vi "Init.vi"(8 "error in (no error)":errorcluster, 9 "Clock type":enum8{"Internal", "External", "PXI"}(ring), 10 "Slot":u16) -> (0 "error out":errorcluster, 3 "MagiQmw3 out":refnum<class "MagiQmw3.lvclass">)   [LabVIEW 2010, in "MagiQmw3.lvclass"]
uses:
  MagiQmw3.lvclass
panel:
  out "path":path
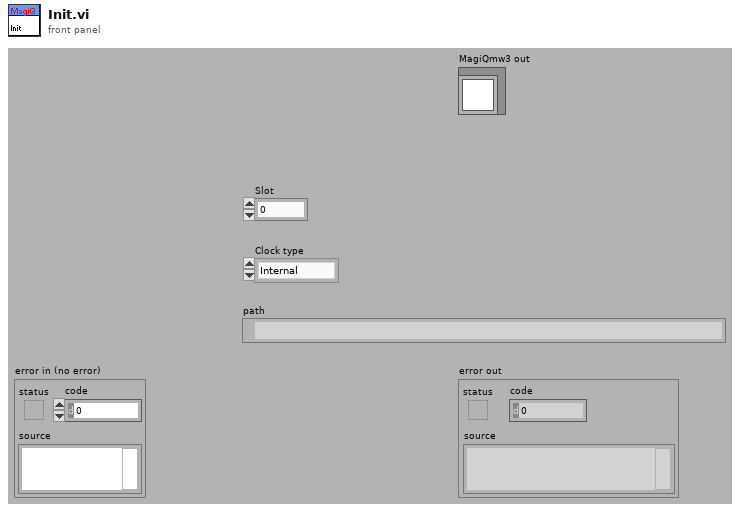
[diagram p1: front panel]
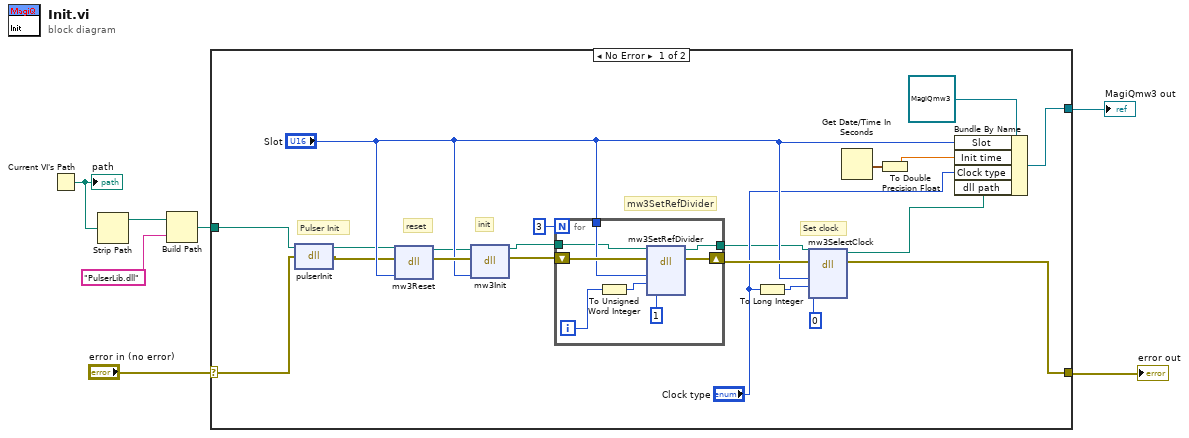
[diagram p0: block diagram]
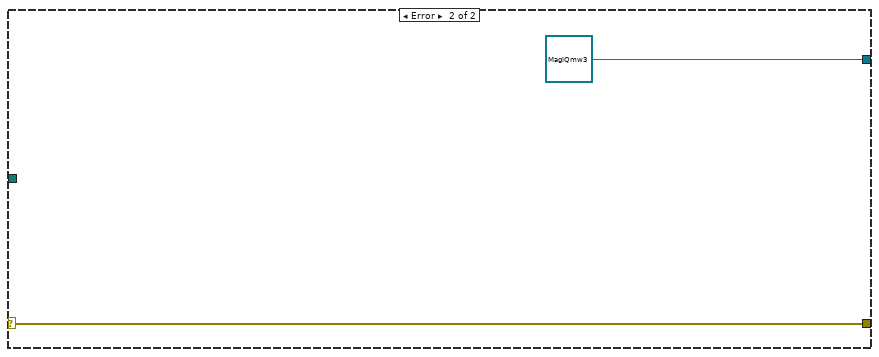
[diagram p2: hidden frame]
diagram:
  n1 = Current VI's Path() -> (path=w4:path)
  "path" <- w4
  n2 = Strip Path(path=w4) -> (stripped path=w3:path)  [unwired: 1 out]
  n3 = Build Path(base path=w3, name or relative path="PulserLib.dll") -> (appended path=w1:path)
  n4 = case shown="No Error" "error in (no error)" {
    selector: "error in (no error)" -> [w9 w38]
    tunnel: [w19 w38] -> w6
    tunnel: [w28 refnum<class "MagiQmw3.lvclass"> refnum ("MagiQmw3 in")] -> w5
    tunnel: w1 -> [w11 _]
    frame No Error {
      # "Pulser Init"
      # "Set clock"
      # "mw3SetRefDivider"
      # "reset"
      # "init"
      n5 = dll-call lib="C:/Documents and Settings/Administrator/My Documents/VIs/magiq/PulserLib.dll" fn="pulserInit"(path in=w11, error in=w9) -> (path out=w10:path, error out=w8:errorcluster)  [unwired: 2 in]
      n6 = dll-call lib="PulserLib.dll" fn="mw3Reset"(path in=w10, error in=w8, "slot"="Slot") -> (path out=w15:path, error out=w24:errorcluster)  [unwired: 3 in]
      n7 = dll-call lib="PulserLib.dll" fn="mw3Init"(path in=w15, error in=w24, "slot"="Slot") -> (path out=w14:path, error out=w22:errorcluster)  [unwired: 3 in]
      n8 = for {
        N: 3 -> [_]
        shift-right: [w36] -> w21
        shift-left: w22 -> [w34]
        tunnel: "Slot" -> [w31]
        tunnel: w14 -> [w30]
        tunnel: [w29] -> w13
        i -> [w32]
        n9 = To Unsigned Word Integer(number=w32) -> (unsigned 16bit integer=w33:u16)
        n10 = dll-call lib="PulserLib.dll" fn="mw3SetRefDivider"(path in=w30, error in=w34, "slot"=w31, "ch"=w33, "val"=u64 1) -> (path out=w29:path, error out=w36:errorcluster)  [unwired: 5 in]
      }
      n11 = To Long Integer(number="Clock type") -> (32bit integer=w18:i32)
      n12 = dll-call lib="PulserLib.dll" fn="mw3SelectClock"(path in=w13, error in=w21, "slot"="Slot", "clockType"=w18, "clkMhz"=u64 0) -> (path out=w12:path, error out=w19:errorcluster)  [unwired: 5 in]
      n13 = Get Date/Time In Seconds() -> (seconds since 1Jan1904=w27:timestamp)
      n14 = To Double Precision Float(number=w27) -> (double precision float=w26:dbl)
      n15 = Bundle By Name(cluster=refnum<class "MagiQmw3.lvclass"> refnum ("MagiQmw3 in"), "Slot"="Slot", "Init time"=w26, "Clock type"="Clock type", "dll path"=w12) -> (w28:refnum<class "MagiQmw3.lvclass">)
    }
    frame Error {
    }
  }
  "error out" <- w6
  "MagiQmw3 out" <- w5
